vi "提取仪器参数 (子VI).vi"(10 "因子编码":string, 11 "数据输入":string[](array[string])) -> (3 "字符串":string)   [LabVIEW 2016, in "数据传输系统-02.lvlib"]
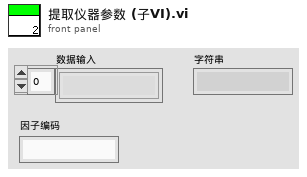
[diagram p1: front panel]
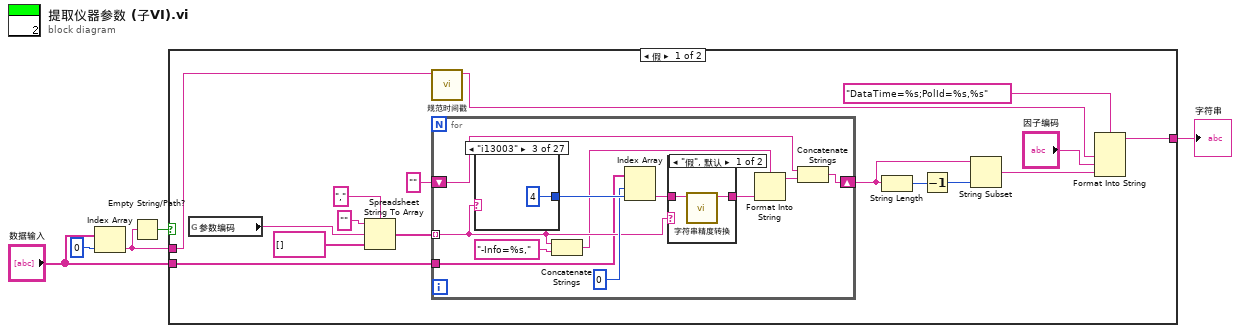
[diagram p0: block diagram]
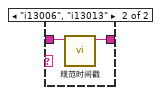
[diagram p2: hidden frame]
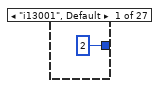
[diagram p3: hidden frame]
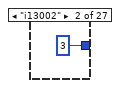
[diagram p4: hidden frame]
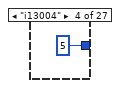
[diagram p5: hidden frame]
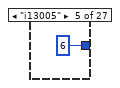
[diagram p6: hidden frame]
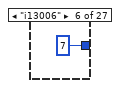
[diagram p7: hidden frame]
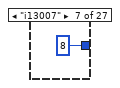
[diagram p8: hidden frame]
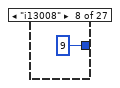
[diagram p9: hidden frame]
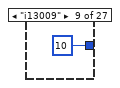
[diagram p10: hidden frame]
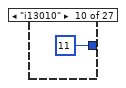
[diagram p11: hidden frame]
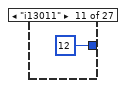
[diagram p12: hidden frame]
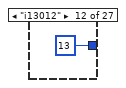
[diagram p13: hidden frame]
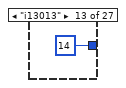
[diagram p14: hidden frame]
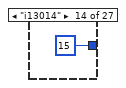
[diagram p15: hidden frame]
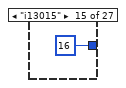
[diagram p16: hidden frame]
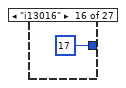
[diagram p17: hidden frame]
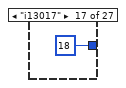
[diagram p18: hidden frame]
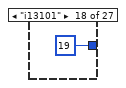
[diagram p19: hidden frame]
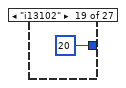
[diagram p20: hidden frame]
diagram:
  n1 = Index Array(array="数据输入", index=0 ("索引")) -> (element=w2:string)
  n2 = Empty String/Path?(string/path=w2) -> (empty?=w3:bool)
  n3 = case shown="假" w3 {
    tunnel: [w10 ""] -> w5
    tunnel: "数据输入" -> [w7 _]
    tunnel: w2 -> [w6 _]
    frame False {
      n4 = global read "全局 提取仪器参数.vi" "参数编码"() -> (w18:string)
      n5 = Spreadsheet String To Array(delimiter (Tab)="," ("分隔符(Tab)"), format string="" ("格式字符串"), spreadsheet string=w18, array type (2D Dbl)=string[] []) -> (array=w16:string[])
      n6 = call "规范时间戳.vi"("字符串"=w6) -> ("result string"=w9:string)  [unwired: 10 in]
      n7 = for {
        shift-right: [w28] -> w14
        shift-left: "" -> [w27]
        tunnel: w16 -> [w29] mode=indexing
        tunnel: w7 -> [w25]
        n8 = case shown="\"i13003\"" w29 {
          tunnel: [2 ("索引") 3 ("索引") 4 ("索引") 5 ("索引") 6 ("索引") 7 ("索引") 8 ("索引") 9 ("索引") 10 ("索引") 11 ("索引") 12 ("索引") 13 ("索引") 14 ("索引") 15 ("索引") 16 ("索引") 17 ("索引") 18 ("索引") 19 ("索引") 20 ("索引") 21 ("索引") 22 ("索引") 23 ("索引") 24 ("索引") 25 ("索引") 26 ("索引") 27 ("索引") 28 ("索引")] -> w32
          frame "i13001", Default {
          }
          frame "i13002" {
          }
          frame "i13003" {
          }
          frame "i13004" {
          }
          frame "i13005" {
          }
          frame "i13006" {
          }
          frame "i13007" {
          }
          frame "i13008" {
          }
          frame "i13009" {
          }
          frame "i13010" {
          }
          frame "i13011" {
          }
          frame "i13012" {
          }
          frame "i13013" {
          }
          frame "i13014" {
          }
          frame "i13015" {
          }
          frame "i13016" {
          }
          frame "i13017" {
          }
          frame "i13101" {
          }
          frame "i13102" {
          }
          frame "i13103" {
          }
          frame "i13104" {
          }
          frame "i13105" {
          }
          frame "i13106" {
          }
          frame "i13107" {
          }
          frame "i13108" {
          }
          frame "i13109" {
          }
          frame "i13110" {
          }
        }
        n9 = Concatenate Strings(w29, "-Info=%s," ("格式字符串")) -> (w23:string)
        n10 = Index Array(array=w25, index #1=0 ("索引"), index #2=w32) -> (element #2=w30:string)  [unwired: 1 out]
        n11 = case shown="\"假\", 默认" w29 {
          tunnel: w30 -> [w34 w36]
          tunnel: [w33 w35] -> w22
          frame "假", Default {
            n12 = call "字符串精度转换.vi"("输入字符串"=w34) -> ("输出字符串"=w33:string)  [unwired: 9 in, 1 out]
          }
          frame "i13006", "i13013" {
            n13 = call "规范时间戳.vi"("字符串"=w36) -> ("result string"=w35:string)  [unwired: 10 in]
          }
        }
        n14 = Format Into String(format string=w23, w22) -> (resulting string=w26:string)  [unwired: 2 in, 1 out]
        n15 = Concatenate Strings(w27, w26) -> (w28:string)
      }
      n16 = String Length(string=w14) -> (length=w13:i32)
      n17 = Decrement(x=w13) -> (x-1=w12:i32)
      n18 = String Subset(string=w14, length (rest)=w12) -> (substring=w11:string)  [unwired: 1 in]
      n19 = Format Into String(format string="DataTime=%s;PolId=%s,%s" ("格式字符串"), w9, "因子编码", w11) -> (resulting string=w10:string)  [unwired: 2 in, 1 out]
    }
    frame True {
    }
  }
  "字符串" <- w5
